vi "ConvertRTPCBytes.vi"(1 "Device Input Cluster":T1={"Dnet"="", "Node"=0, "Type"="", "ID Number"=0, "SCCM"=0.0, "FullScale"=0.0, "Input Bytes"=0, "Output Bytes"=0, "Input Start Location"=0, "Output Start Location"=0, "Enabled"=TRUE, "Bytes"=[]}) -> (0 "Device Output Cluster":T1={"Dnet"="", "Node"=0, "Type"="", "ID Number"=0, "SCCM"=0.0, "FullScale"=0.0, "Input Bytes"=0, "Output Bytes"=0, "Input Start Location"=0, "Output Start Location"=0, "Enabled"=TRUE, "Bytes"=[]})   [LabVIEW 2011]
uses:
  Excel/Device Cluster.ctl
  GlobalVariables.vi
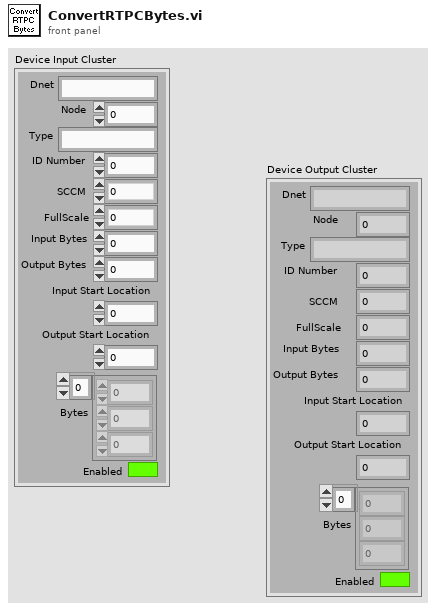
[diagram p1: front panel]
types:
  T1 = typedef "Device Cluster.ctl" = cluster{"Dnet":string, "Node":i32, "Type":string, "ID Number":u8, "SCCM":dbl, "FullScale":dbl, "Input Bytes":i32, "Output Bytes":i32, "Input Start Location":i32, "Output Start Location":i32, "Enabled":bool, "Bytes":u8[]}
  T2 = cluster{"[0]":u8, "[1]":u8, "[2]":u8, "[3]":u8, "[4]":u8, "[5]":u8, "[6]":u8, "[7]":u8}
  T3 = typedef "RTPC Cluster.ctl" = cluster{"ID Number":u8, "Status":bool[], "Flow (SCCM)":dbl, "Pressure (SCCM)":dbl, "Valve":i16, "Active Instance":i8, "Output":dbl}
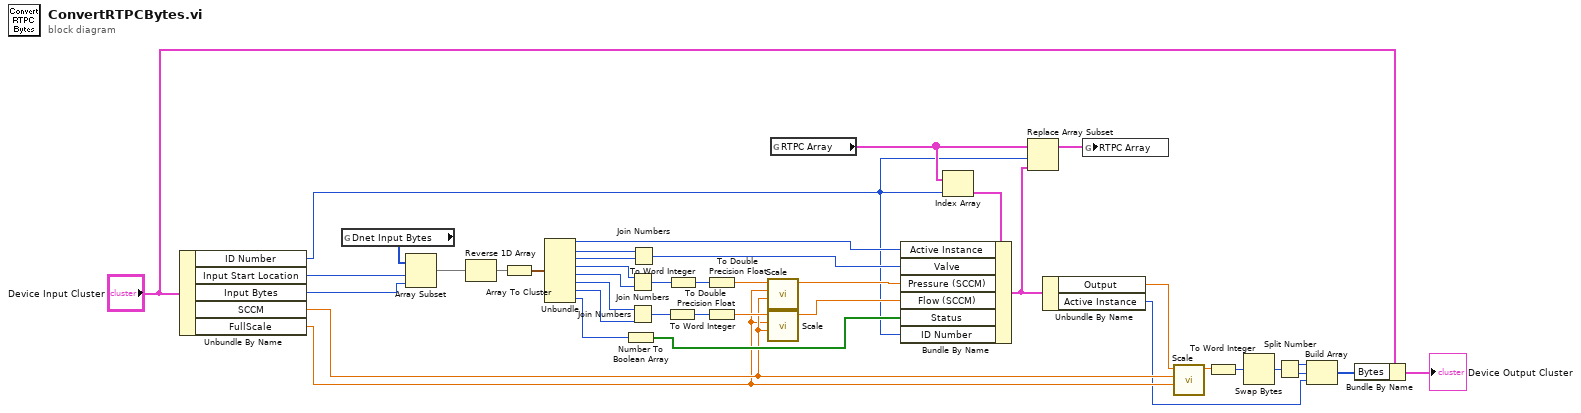
[diagram p0: block diagram]
diagram:
  n1 = Unbundle By Name("Device Input Cluster") -> ("ID Number"=w7:u8, "Input Start Location"=w26:i32, "Input Bytes"=w27:i32, "SCCM"=w5:dbl, "FullScale"=w4:dbl)
  n2 = global read "GlobalVariables.vi" "Dnet Input Bytes"() -> (w29:u8[])
  n3 = Array Subset(array=w29, index=w26, length=w27) -> (w28:u8[])
  n4 = Reverse 1D Array(array=w28) -> (reversed array=w30:u8[])
  n5 = Array To Cluster(array=w30) -> (cluster=w25:T2)
  n6 = Unbundle(w25) -> ("[0]"=w19:u8, "[1]"=w31:u8, "[2]"=w32:u8, "[3]"=w37:u8, "[4]"=w38:u8, "[5]"=w39:u8, "[6]"=w40:u8, "[7]"=w41:u8)
  n7 = Number To Boolean Array(number=w41) -> (Boolean array=w18:bool[])
  n8 = Join Numbers(hi=w37, lo=w38) -> ((hi.lo)=w33:u16)
  n9 = Join Numbers(hi=w39, lo=w40) -> ((hi.lo)=w34:u16)
  n10 = Join Numbers(hi=w31, lo=w32) -> ((hi.lo)=w20:u16)
  n11 = To Word Integer(number=w34) -> (16bit integer=w35:i16)
  n12 = To Word Integer(number=w33) -> (16bit integer=w36:i16)
  n13 = To Double Precision Float(number=w36) -> (double precision float=w24:dbl)
  n14 = To Double Precision Float(number=w35) -> (double precision float=w23:dbl)
  n15 = call "Scale.vi"("Factor"=w5, "FullScale"=w4, "Input"=w24) -> ("Output"=w22:dbl)  [unwired: 8 in]
  n16 = call "Scale.vi"("Factor"=w5, "FullScale"=w4, "Input"=w23) -> ("Output"=w21:dbl)  [unwired: 8 in]
  n17 = global read "GlobalVariables.vi" "RTPC Array"() -> (w10:T3[])
  n18 = Index Array(array=w10, index=w7) -> (element=w8:T3)
  n19 = Bundle By Name(cluster=w8, "Active Instance"=w19, "Valve"=w20, "Pressure (SCCM)"=w22, "Flow (SCCM)"=w21, "Status"=w18, "ID Number"=w7) -> (w2:T3)
  n20 = Replace Array Subset(array=w10, new element=w2, index=w7) -> (w9:T3[])
  n21 = Unbundle By Name(w2) -> ("Output"=w6:dbl, "Active Instance"=w1:i8)
  n22 = global write "GlobalVariables.vi" "RTPC Array"(w9) -> ()
  n23 = call "Scale.vi"("Factor"=w4, "FullScale"=w5, "Input"=w6) -> ("Output"=w17:dbl)  [unwired: 8 in]
  n24 = To Word Integer(number=w17) -> (16bit integer=w16:i16)
  n25 = Swap Bytes(anything=w16) -> (byte swapped=w15:i16)
  n26 = Split Number(x=w15) -> (hi(x)=w13:u8, lo(x)=w14:u8)
  n27 = Build Array(w13, w14, w1) -> (w11:u8[])
  n28 = Bundle By Name(cluster="Device Input Cluster", "Bytes"=w11) -> (→"Device Output Cluster":T1)
